vi "Inst.Transport.CallByReference.vi"(8 "error in (no error)":errorcluster, 9 "VI":T1=enum."LockinTimeDelay", 10 "vi path":path, 11 "Transport":refnum<class "Transport.lvclass">) -> (0 "error out":errorcluster)   [LabVIEW 2019, in "Inst.Transport.lvclass"]
uses:
  Inst.Transport.lvclass
  Transport/Transport.lvclass
  Typedefs/Inst.Transport.Methods--Enum.ctl
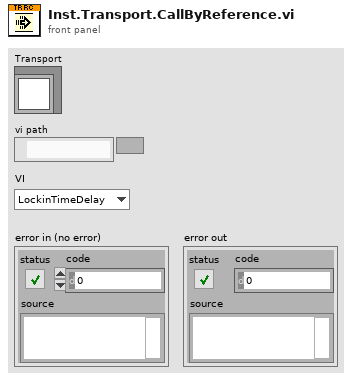
[diagram p1: front panel]
types:
  T1 = typedef "Inst.Transport.lvclass/Inst.Transport.Methods--Enum.ctl" = enum16{"LockinSweep", "LockinTime", "LockinTimeDelay"}
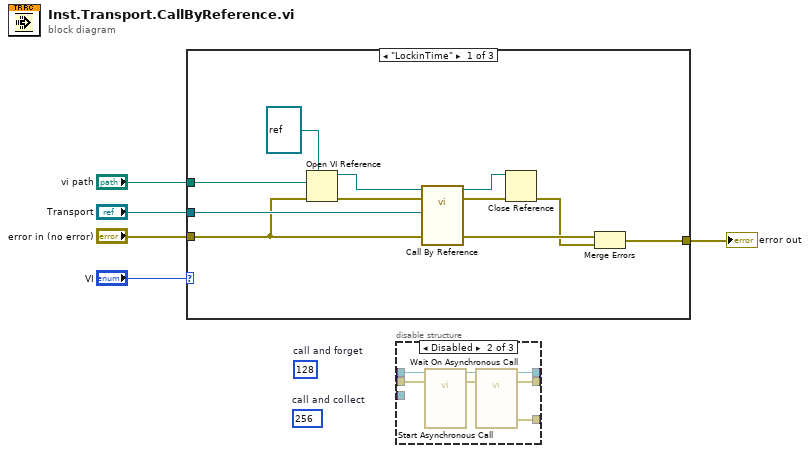
[diagram p0: block diagram]
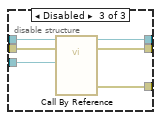
[diagram p3: hidden frame]
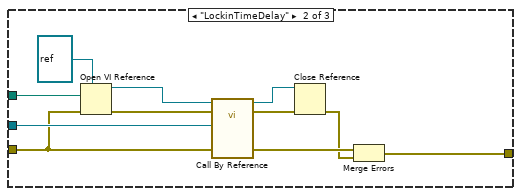
[diagram p4: hidden frame]
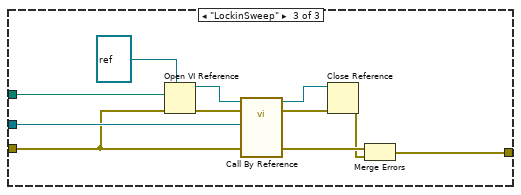
[diagram p5: hidden frame]
diagram:
  (unwired) 256  # call and collect
  (unwired) 128  # call and forget
  n1 = case shown="\"LockinTime\"" "VI" {
    tunnel: "vi path" -> [w14 w25 w38]
    tunnel: "Transport" -> [w12 w23 w37]
    tunnel: [w7 w18 w36] -> w1
    tunnel: "error in (no error)" -> [w6 w17 w28]
    frame "LockinTime" {
      n2 = Open VI Reference(type specifier VI Refnum (for type only)=refnum<vi> refnum, vi path=w14, error in (no error)=w6) -> (vi reference=w13:refnum<vi>, error out=w15:errorcluster)  [unwired: 3 in]
      n3 = call-by-ref "?"(reference=w13, error in=w15, 8:"error in (no error)"=w6, "Transport"=w12) -> (reference out=w10:refnum<vi>, error out=w11:errorcluster, 0:"error out"=w9:errorcluster)  [unwired: 8 in, 1 out]
      n4 = Close Reference(reference=w10, error in (no error)=w11) -> (error out=w8:errorcluster)
      n5 = Merge Errors(w9, w8) -> (w7:errorcluster)
    }
    frame "LockinTimeDelay" {
      n6 = Open VI Reference(type specifier VI Refnum (for type only)=refnum<vi> refnum, vi path=w25, error in (no error)=w17) -> (vi reference=w24:refnum<vi>, error out=w26:errorcluster)  [unwired: 3 in]
      n7 = call-by-ref "?"(reference=w24, error in=w26, 8:"error in (no error)"=w17, "Transport"=w23) -> (reference out=w22:refnum<vi>, error out=w21:errorcluster, 0:"error out"=w20:errorcluster)  [unwired: 8 in, 1 out]
      n8 = Close Reference(reference=w22, error in (no error)=w21) -> (error out=w19:errorcluster)
      n9 = Merge Errors(w20, w19) -> (w18:errorcluster)
    }
    frame "LockinSweep" {
      n10 = Open VI Reference(type specifier VI Refnum (for type only)=refnum<vi> refnum, vi path=w38, error in (no error)=w28) -> (vi reference=w35:refnum<vi>, error out=w30:errorcluster)  [unwired: 3 in]
      n11 = call-by-ref "?"(reference=w35, error in=w30, "Transport"=w37, 3:"error in (no error)"=w28) -> (reference out=w33:refnum<vi>, error out=w29:errorcluster, 10:"error out"=w32:errorcluster)  [unwired: 7 in, 1 out]
      n12 = Close Reference(reference=w33, error in (no error)=w29) -> (error out=w31:errorcluster)
      n13 = Merge Errors(w32, w31) -> (w36:errorcluster)
    }
  }
  "error out" <- w1
  n14 = disable-structure shown="Disabled" {
    disable-tunnel: _ -> [_ w45 w48]
    disable-tunnel: [_ w42 w49] -> _
    disable-tunnel: _ -> [_ w41 w51]
    disable-tunnel: [_ w40 w50] -> _
    disable-tunnel: _ -> [_ _ w47]
    disable-tunnel: [_ w39 w46] -> _
    frame Enabled {
    }
    frame Disabled {
      n15 = call-by-ref "Start Asynchronous Call"(reference=w41, error in=w45) -> (reference out=w44:refnum<vi>, error out=w43:errorcluster)  [unwired: 10 in, 2 out]
      n16 = call-by-ref "Wait On Asynchronous Call"(reference=w44, error in=w43) -> (reference out=w40:refnum<vi>, error out=w42:errorcluster, 0:"error out"=w39:errorcluster)  [unwired: 10 in, 1 out]
    }
    frame Disabled {
      n17 = call-by-ref "?"(reference=w51, error in=w48, "Transport"=w47) -> (reference out=w50:refnum<vi>, error out=w49:errorcluster, 0:"error out"=w46:errorcluster)  [unwired: 9 in, 1 out]
    }
  }
